vi "Titel-Text aus Bildtasten.vi"(6 "Tasten-Index":i32, 11 "Referenz Bildtasten":refnum<vi>) -> (3 "Titel-Text":string)   [LabVIEW 2020, in "Bildwechsel.lvlib"]
uses:
  Bildwechsel.lvlib
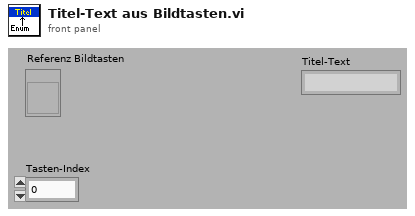
[diagram p1: front panel]
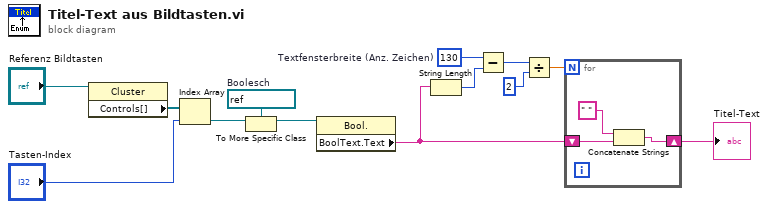
[diagram p0: block diagram]
diagram:
  w6 = 130  # Textfensterbreite (Anz. Zeichen)
  w12 = refnum<vi> refnum  # Boolesch
  n1 = property class="Cluster"(reference="Referenz Bildtasten") -> ("Controls[]"=w8:refnum<vi>[])  [unwired: 1 in, 2 out]
  n2 = Index Array(array=w8, index="Tasten-Index") -> (element=w11:refnum<vi>)
  n3 = To More Specific Class(target class=w12, reference=w11) -> (specific class reference=w13:refnum<vi>)  [unwired: 1 in, 1 out]
  n4 = property class="Bool."(reference=w13) -> ("BoolText.Text"=w2:string)  [unwired: 1 in, 2 out]
  n5 = String Length(string=w2) -> (length=w7:i32)
  n6 = Subtract(x=w6, y=w7) -> (x-y=w5:i32)
  n7 = Divide(x=w5, y=2) -> (x/y=w3:dbl)
  n8 = for {
    N: w3 -> [_]
    shift-right: [w14] -> w1
    shift-left: w2 -> [w16]
    n9 = Concatenate Strings(" " ("String"), w16) -> (w14:string)
  }
  "Titel-Text" <- w1
